vi "Trim_Filename.vi"(1 "Input string":string, 2 "length":i32=22) -> (0 "output string":string)   [LabVIEW 2025]
doc: "Trim the input filename into a 22-character limit string.\nThe filename has to start with a letter and contains good characters only.\n^[a-zA-Z]+[a-zA-Z0-9 +&=-_#$@.,]*\nAuthor: Scott Hannahs <sth@magnet.fsu.edu>\n\nThis software is licensed for use under the “MIT License\"\nCopyright (c) 2025 Scott Hannahs, sth@sth@magnet.sthnet.net\n\nPermission is hereby granted, free of charge, to any person obtaining a copy of this software and associated documentation files (the \"Software\"), to deal in the Software without restriction, including without limitation the rights to use, copy, modify, merge, publish, distribute, sublicense, and/or sell copies of the Software, and to permit persons to whom the Software is furnished to do so, subject to the following conditions: The above copyright notice and this permission notice shall be included in all copies or substantial portions of the Software.\n\nTHE SOFTWARE IS PROVIDED \"AS IS\", WITHOUT WARRANTY OF ANY KIND, EXPRESS OR IMPLIED, INCLUDING BUT NOT LIMITED TO THE WARRANTIES OF MERCHANTABILITY, FITNESS FOR A PARTICULAR PURPOSE AND NONINFRINGEMENT. IN NO EVENT SHALL THE AUTHORS OR COPYRIGHT HOLDERS BE LIABLE FOR ANY CLAIM, DAMAGES OR OTHER LIABILITY, WHETHER IN AN ACTION OF CONTRACT, TORT OR OTHERWISE, ARISING FROM, OUT OF OR IN CONNECTION WITH THE SOFTWARE OR THE USE OR OTHER DEALINGS IN THE SOFTWARE."
panel:
  out "after substring":string
  out "before substring":string
  out "match substring":string
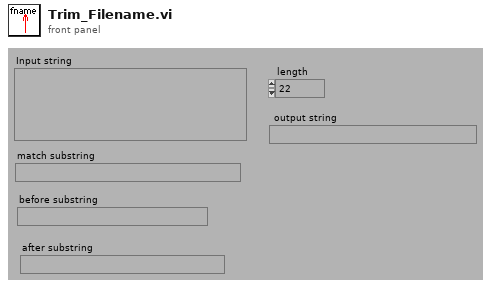
[diagram p1: front panel]
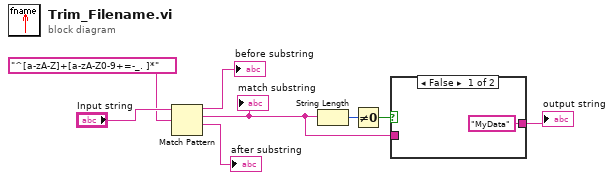
[diagram p0: block diagram]
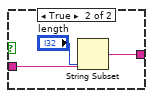
[diagram p2: hidden frame]
diagram:
  n1 = Match Pattern(string="Input string", regular expression="^[a-zA-Z]+[a-zA-Z0-9+=-_. ]*") -> (before substring=→"before substring":string, match substring=w2:string, after substring=→"after substring":string)  [unwired: 1 in, 1 out]
  "match substring" <- w2
  n2 = String Length(string=w2) -> (length=w3:i32)
  n3 = Not Equal To 0?(x=w3) -> (x != 0?=w4:bool)
  n4 = case shown="False" w4 {
    tunnel: w2 -> [_ w12]
    tunnel: ["MyData" w11] -> w1
    frame False {
    }
    frame True {
      n5 = String Subset(string=w12, length (rest)="length") -> (substring=w11:string)  [unwired: 1 in]
    }
  }
  "output string" <- w1
